vi "Serialise Content.vi"(8 "error in (no error)":errorcluster, 11 "object in":refnum<class "Message Class.lvclass">) -> (0 "error out":errorcluster, 2 "Content":string, 3 "object out":refnum<class "Message Class.lvclass">)   [LabVIEW 2018, in "ClientMessaging.lvlib" / "Message Class.lvclass"]
doc: "Serialise the content attribute"
uses:
  Message Class.lvclass
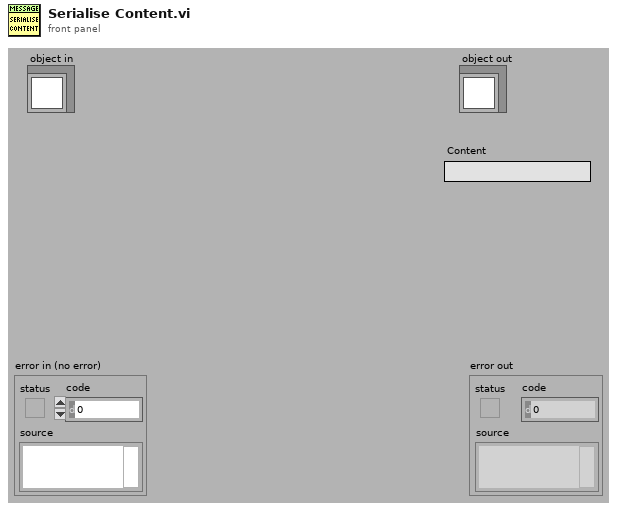
[diagram p1: front panel]
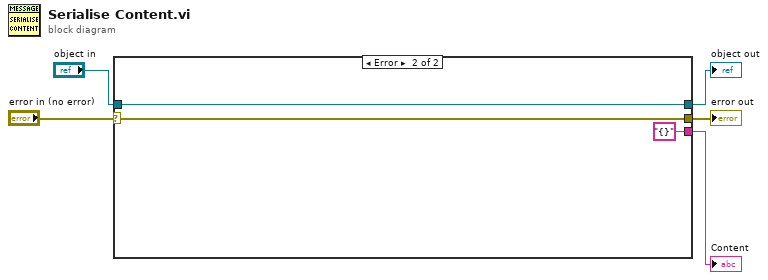
[diagram p0: block diagram]
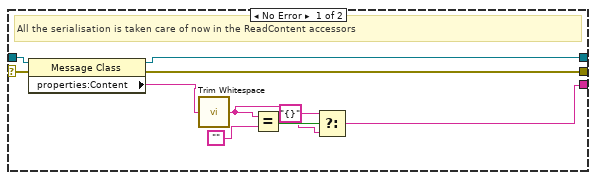
[diagram p2: hidden frame]
diagram:
  n1 = case shown="Error" "error in (no error)" {
    selector: "error in (no error)" -> [w13 w18]
    tunnel: [w12 w18] -> w4
    tunnel: [w14 w17] -> w2
    tunnel: "object in" -> [w15 w17]
    tunnel: [w6 "{}" ("trimmed string")] -> w1
    frame No Error {
      # "All the serialisation is taken care of now in the ReadContent accessors"
      n2 = property class="Message Class"(reference=w15, error in=w13) -> (reference out=w14:refnum<class "Message Class.lvclass">, error out=w12:errorcluster, "properties:Content"=w11:string)
      n3 = call <vilib>:"Trim Whitespace.vi"("string"=w11) -> ("trimmed string"=w8:string)  [unwired: 1 in]
      n4 = Equal?(x=w8, y="") -> (x = y?=w9:bool)
      n5 = Select(t="{}", s=w9, f=w8) -> (s? t:f=w6:string)
    }
    frame Error {
    }
  }
  "error out" <- w4
  "object out" <- w2
  "Content" <- w1
